vi "Selection Mode To Browse Options.vi"(11 "Selection Mode":T1) -> (1 "Treat LLB's as Folders":bool, 2 "New or Existing":T2, 3 "Files or Folders":T3)   [LabVIEW 2018, in "Path Data Type.lvclass"]
uses:
  Path Data Type.lvclass
  Files or Folders.ctl
  New or Existing.ctl
  Selection Mode.ctl
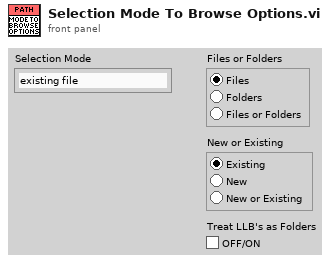
[diagram p1: front panel]
types:
  T1 = typedef "Path Data Type.lvclass/Selection Mode.ctl" = enum32{"existing file", "new file", "new or existing file", "existing dir", "new dir", "new or existing dir", "existing file (use LLBs)", "new file (use LLBs)", "new or existing file (use LLBs)", "new or existing file or directory (use LLBs)", "existing dir (use LLBs)", "new dir (use LLBs)", "new or existing dir (use LLBs)", "existing file or dir", "new file or dir", "new or existing file or dir", "existing file or dir (use LLBs)", "new file or dir (use LLBs)"}
  T2 = typedef "Path Data Type.lvclass/New or Existing.ctl" = enum32{"Existing", "New", "New or Existing"}
  T3 = typedef "Path Data Type.lvclass/Files or Folders.ctl" = enum32{"Files", "Folders", "Files or Folders"}
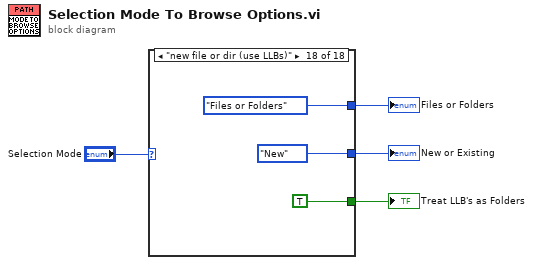
[diagram p0: block diagram]
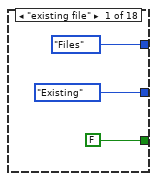
[diagram p2: hidden frame]
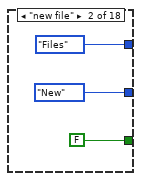
[diagram p3: hidden frame]
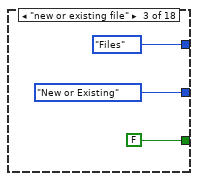
[diagram p4: hidden frame]
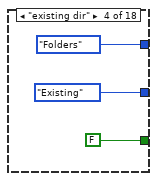
[diagram p5: hidden frame]
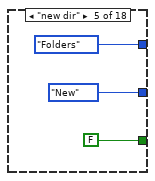
[diagram p6: hidden frame]
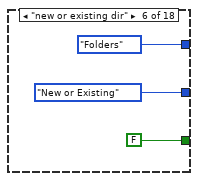
[diagram p7: hidden frame]
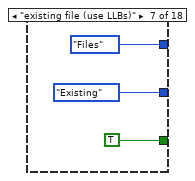
[diagram p8: hidden frame]
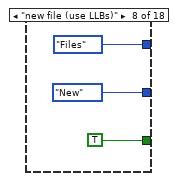
[diagram p9: hidden frame]
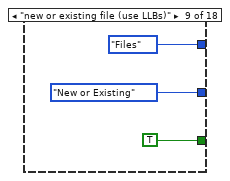
[diagram p10: hidden frame]
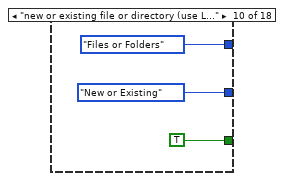
[diagram p11: hidden frame]
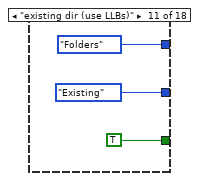
[diagram p12: hidden frame]
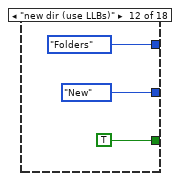
[diagram p13: hidden frame]
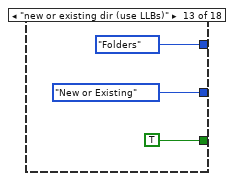
[diagram p14: hidden frame]
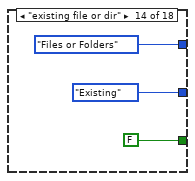
[diagram p15: hidden frame]
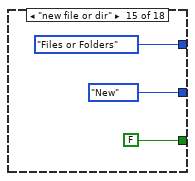
[diagram p16: hidden frame]
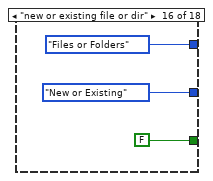
[diagram p17: hidden frame]
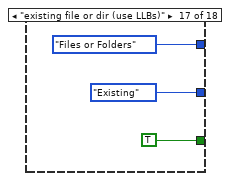
[diagram p18: hidden frame]
diagram:
  n1 = case shown="\"new file or dir (use LLBs)\"" "Selection Mode" {
    tunnel: [Files_or_Folders."Files" ("Files or Folders") Files_or_Folders."Files" ("Files or Folders") Files_or_Folders."Files" ("Files or Folders") Files_or_Folders."Folders" ("Files or Folders") Files_or_Folders."Folders" ("Files or Folders") Files_or_Folders."Folders" ("Files or Folders") Files_or_Folders."Files" ("Files or Folders") Files_or_Folders."Files" ("Files or Folders") Files_or_Folders."Files" ("Files or Folders") Files_or_Folders."Files or Folders" ("Files or Folders") Files_or_Folders."Folders" ("Files or Folders") Files_or_Folders."Folders" ("Files or Folders") Files_or_Folders."Folders" ("Files or Folders") Files_or_Folders."Files or Folders" ("Files or Folders") Files_or_Folders."Files or Folders" ("Files or Folders") Files_or_Folders."Files or Folders" ("Files or Folders") Files_or_Folders."Files or Folders" ("Files or Folders") Files_or_Folders."Files or Folders" ("Files or Folders")] -> w4
    tunnel: [New_or_Existing."Existing" ("New or Existing") New_or_Existing."New" ("New or Existing") New_or_Existing."New or Existing" ("New or Existing") New_or_Existing."Existing" ("New or Existing") New_or_Existing."New" ("New or Existing") New_or_Existing."New or Existing" ("New or Existing") New_or_Existing."Existing" ("New or Existing") New_or_Existing."New" ("New or Existing") New_or_Existing."New or Existing" ("New or Existing") New_or_Existing."New or Existing" ("New or Existing") New_or_Existing."Existing" ("New or Existing") New_or_Existing."New" ("New or Existing") New_or_Existing."New or Existing" ("New or Existing") New_or_Existing."Existing" ("New or Existing") New_or_Existing."New" ("New or Existing") New_or_Existing."New or Existing" ("New or Existing") New_or_Existing."Existing" ("New or Existing") New_or_Existing."New" ("New or Existing")] -> w2
    tunnel: [FALSE FALSE FALSE FALSE FALSE FALSE TRUE TRUE TRUE TRUE TRUE TRUE TRUE FALSE FALSE FALSE TRUE TRUE] -> w1
    frame "existing file" {
    }
    frame "new file" {
    }
    frame "new or existing file" {
    }
    frame "existing dir" {
    }
    frame "new dir" {
    }
    frame "new or existing dir" {
    }
    frame "existing file (use LLBs)" {
    }
    frame "new file (use LLBs)" {
    }
    frame "new or existing file (use LLBs)" {
    }
    frame "new or existing file or directory (use LLBs)" {
    }
    frame "existing dir (use LLBs)" {
    }
    frame "new dir (use LLBs)" {
    }
    frame "new or existing dir (use LLBs)" {
    }
    frame "existing file or dir" {
    }
    frame "new file or dir" {
    }
    frame "new or existing file or dir" {
    }
    frame "existing file or dir (use LLBs)" {
    }
    frame "new file or dir (use LLBs)" {
    }
  }
  "Files or Folders" <- w4
  "New or Existing" <- w2
  "Treat LLB's as Folders" <- w1
